vi "tool_Unicode_Convert ASCII to Unicode (Scalar).vi"(4 "ASCII":string) -> (1 "Unicode":string)   [LabVIEW 2020]
uses:
  kernel32.dll
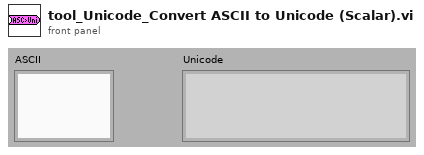
[diagram p1: front panel]
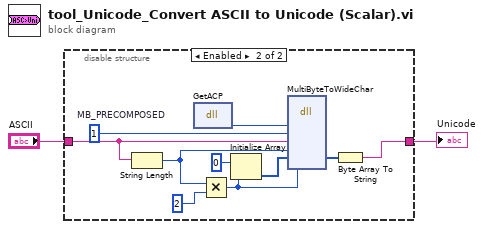
[diagram p0: block diagram]
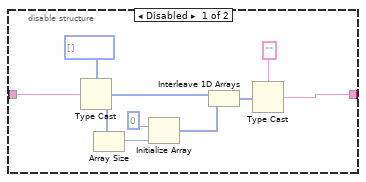
[diagram p2: hidden frame]
diagram:
  n1 = disable-structure shown="Enabled" {
    disable-tunnel: "ASCII" -> [w11 w14]
    disable-tunnel: [w3 w13] -> w1
    frame Disabled {
      n2 = Type Cast(type=u8[] [], x=w11) -> (*(type *) &x=w7:u8[])
      n3 = Array Size(array=w7) -> (size(s)=w9:i32)
      n4 = Initialize Array(u8 0, w9) -> (w6:u8[])
      n5 = Interleave 1D Arrays(w7, w6) -> (w5:u8[])
      n6 = Type Cast(type="", x=w5) -> (*(type *) &x=w3:string)
    }
    frame Enabled {
      w20 = u32 1  # MB_PRECOMPOSED
      n7 = String Length(string=w14) -> (length=w12:i32)
      n8 = dll-call lib="kernel32.dll" fn="GetACP" label="GetACP()"() -> (w15:u32)  [unwired: 3 in, 2 out]
      n9 = Multiply(x=w12, y=2) -> (x*y=w16:i32)
      n10 = Initialize Array(u8 0, w16) -> (w18:u8[])
      n11 = dll-call lib="kernel32.dll" fn="MultiByteToWideChar"("codePage"=w15, "dwFlags"=w20, "pMultiByteStr"=w14, "cbMultiByte"=w12, "lpWideCharStr"=w18, "cchWideChar"=w16) -> ("lpWideCharStr"=w17:u8[])  [unwired: 8 in, 3 out]
      n12 = Byte Array To String(unsigned byte array=w17) -> (string=w13:string)
    }
  }
  "Unicode" <- w1
